vi "WEBDAV EXAMPLE.vi"() -> ()   [LabVIEW 2016, in "数据传输系统.lvlib" / "update.lvlib"]
uses:
  update.lvlib
  <vilib>/WebDAVClient/Advanced/Multi Event/Request Status.ctl
  WebDAV client/WebDAV client.lvclass
  <vilib>/WebDAVClient/NI_WebDAV.lvlib
panel:
  out "进度":u8(slide) scale=0.0..100.0
  out "error out":errorcluster
  in  "push":bool
  in  "pull":bool
  in  "stop":bool
  in  "local file path":path caption="本地文件路径"
  out "request status":T1
  out "total bytes":u64
  out "bytes completed":u64
  in  "error in (no error)":errorcluster caption="错误输入（无错误）"
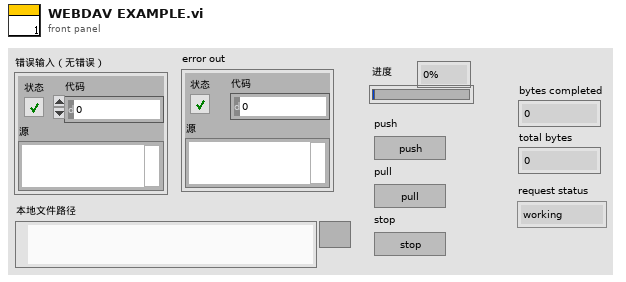
[diagram p1: front panel]
types:
  T1 = typedef "NI_WebDAV.lvlib/Request Status.ctl" = enum16{"working", "complete", "aborted", "timeout", "error"}
  T2 = cluster{"host uri prefix":string, "username":string, "password":string}
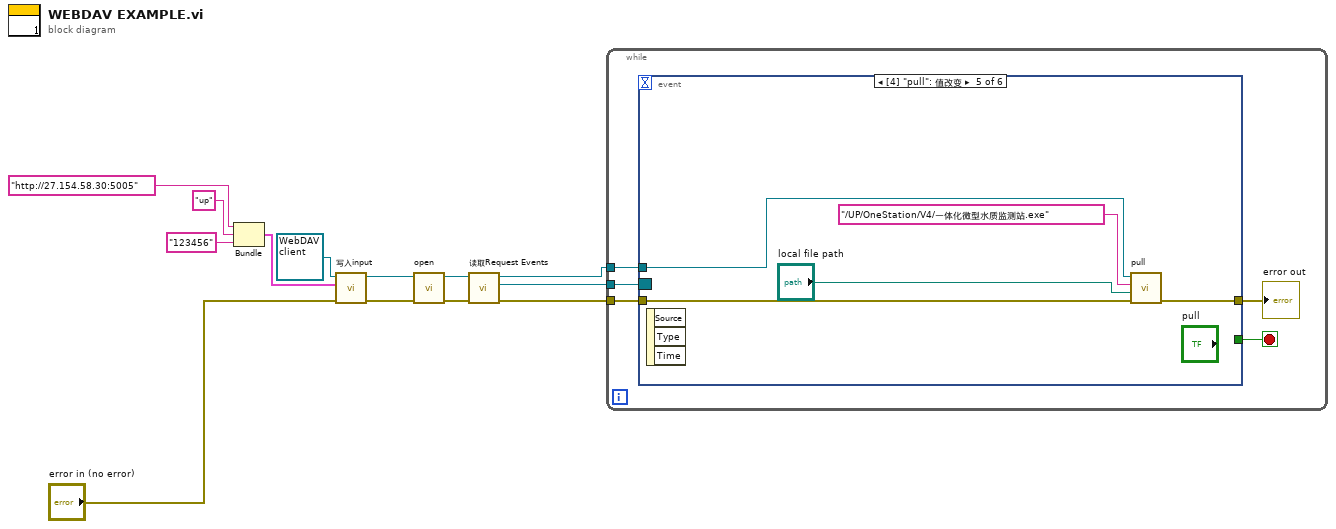
[diagram p0: block diagram]
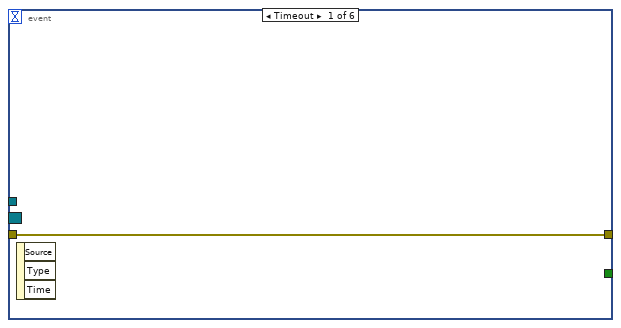
[diagram p2: hidden frame]
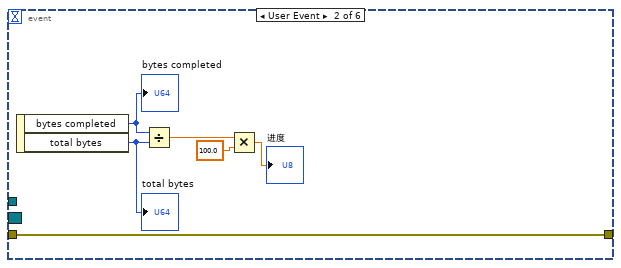
[diagram p3: hidden frame]
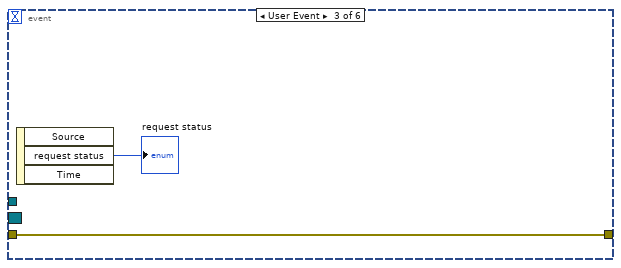
[diagram p4: hidden frame]
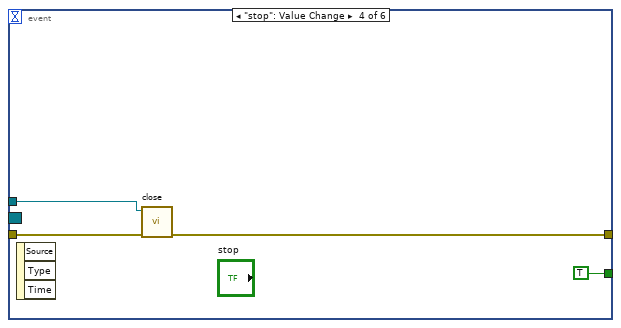
[diagram p5: hidden frame]
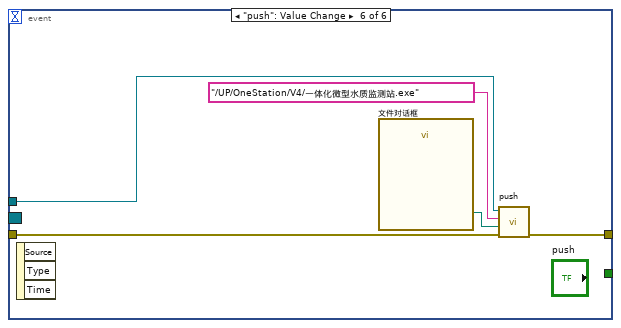
[diagram p6: hidden frame]
diagram:
  n1 = Bundle("host uri prefix"="http://27.154.58.30:5005", "username"="up", "password"="123456") -> (w8:T2)  [unwired: 1 in]
  n2 = call-dynamic "写入input.vi"("error in (no error)"="error in (no error)", "input"=w8, "WebDAV client输入"=refnum<class "WebDAV client.lvclass"> refnum ("update.lvlib:WebDAV client.lvclass")) -> ("error out"=w7:errorcluster, "WebDAV client输出"=w9:refnum<class "WebDAV client.lvclass">)  [unwired: 7 in]
  n3 = call-dynamic "open.vi"("error in (no error)"=w7, "WebDAV client 输入"=w9) -> ("error out"=w5:errorcluster, "WebDAV client 输出"=w4:refnum<class "WebDAV client.lvclass">)  [unwired: 8 in]
  n4 = call-dynamic "读取Request Events.vi"("error in (no error)"=w5, "WebDAV client输入"=w4) -> ("error out"=w3:errorcluster, "Request Events"=w2:refnum<event-registration>, "WebDAV client输出"=w1:refnum<class "WebDAV client.lvclass">)  [unwired: 7 in]
  n5 = while {
    tunnel: w2 -> [w18]
    tunnel: w1 -> [w16]
    tunnel: w3 -> [w15]
    stop <- w17 stop-if-true
    n6 = event shown="[4] \"pull\": 值改变" {
      selector: w18 -> [_ _ _ _ _ _]
      dyn-events: _ -> [_ _ _ _ _ _]
      timeout: _ -> [_ _ _ _ _ _]
      tunnel: [_ _ _ TRUE _ _] -> w17
      tunnel: w16 -> [_ _ _ w30 w36 w41]
      tunnel: w15 -> [w19 w25 w26 w29 w33 w40]
      tunnel: [w19 w25 w26 w28 w32 w39] -> w14
      event Timeout {
        n7 = event-data() -> ()  [unwired: 1 in, 3 out]
      }
      event User Event {
        n8 = event-data() -> ("bytes completed"=w24:u64, "total bytes"=w23:u64)  [unwired: 1 in]
        "bytes completed" <- w24
        "total bytes" <- w23
        n9 = Divide(x=w24, y=w23) -> (x/y=w22:dbl)
        n10 = Multiply(x=w22, y=100.0) -> (x*y=→"进度":dbl)
      }
      event User Event {
        n11 = event-data() -> ("request status"=→"request status":T1)  [unwired: 1 in, 2 out]
      }
      event "stop": Value Change {
        n12 = event-data() -> ()  [unwired: 1 in, 3 out]
        n13 = call-dynamic "close.vi"("error in (no error)"=w29, "WebDAV client 输入"=w30) -> ("error out"=w28:errorcluster)  [unwired: 8 in, 1 out]
      }
      event "pull": Value Change {
        n14 = event-data() -> ()  [unwired: 1 in, 3 out]
        n15 = call-dynamic "pull.vi"("error in (no error)"=w33, "local file path"="local file path", "更新包远端地址"="/UP/OneStation/V4/一体化微型水质监测站.exe", "WebDAV client 输入"=w36) -> ("error out"=w32:errorcluster)  [unwired: 6 in, 1 out]
      }
      event "push": Value Change {
        n16 = event-data() -> ()  [unwired: 1 in, 3 out]
        n17 = call "文件对话框"() -> ("selected path"=w38:path)  [unwired: 12 in, 3 out]
        n18 = call-dynamic "push.vi"("error in (no error)"=w40, "local file path"=w38, "relative uri"="/UP/OneStation/V4/一体化微型水质监测站.exe" ("更新包远端地址"), "WebDAV client 输入"=w41) -> ("error out"=w39:errorcluster)  [unwired: 6 in, 1 out]
      }
    }
    "error out" <- w14
  }
